vi "Array Sizer.vi"(1 "Angular Accelerations":T1 {"Angular \nAccelerations" step=5.0}, 2 "Points out":cluster{"x":dbl, "y":dbl, "th":dbl}[](array[cluster])) -> (0 "output cluster":T1)   [LabVIEW 2019]
panel:
  # "TURN Acceleration"
  # "1"
  # "1"
  # "2"
  # "2"
  # "3"
  # "3"
  # "4"
  # "4"
  # "5"
  # "5"
  # "6"
  # "6"
  # "7"
  # "7"
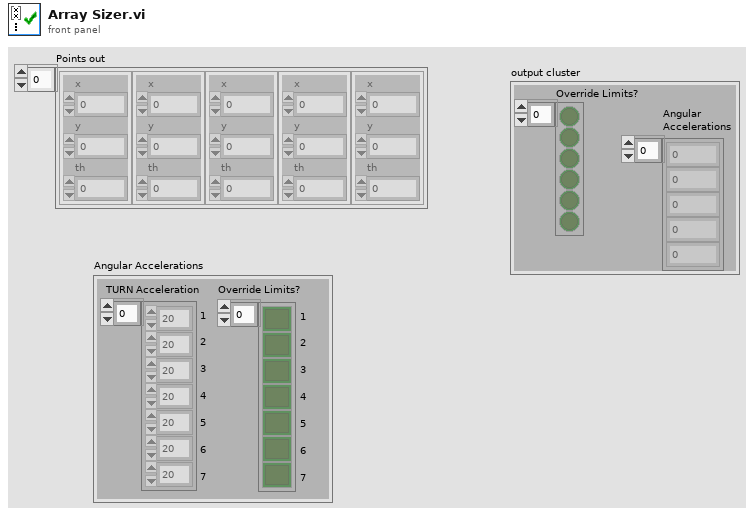
[diagram p1: front panel]
types:
  T1 = cluster{"Angular \nAccelerations":dbl[], "Override Limits?":bool[]}
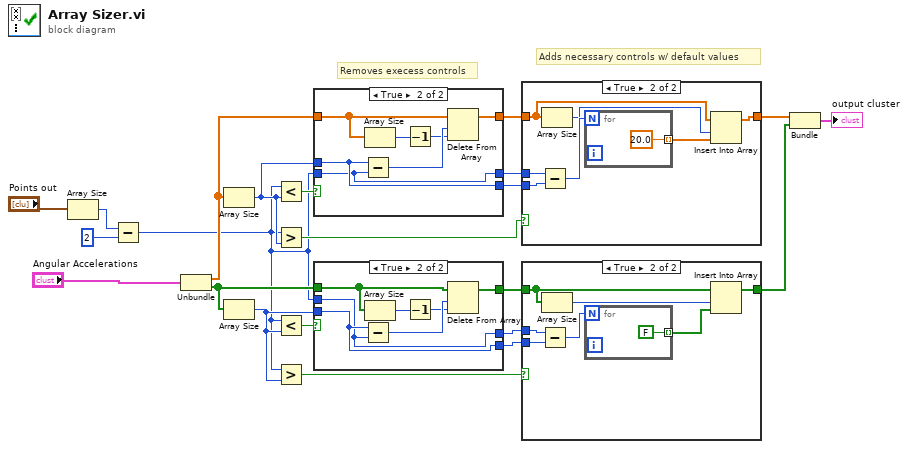
[diagram p0: block diagram]
diagram:
  # "Adds necessary controls w/ default values"
  # "Removes execess controls"
  n1 = Array Size(array="Points out") -> (size(s)=w4:i32)
  n2 = Subtract(x=w4, y=2) -> (x-y=w2:i32)
  n3 = Unbundle("Angular Accelerations") -> ("Angular \nAccelerations"=w18:dbl[], "Override Limits?"=w11:bool[])
  n4 = Array Size(array=w18) -> (size(s)=w17:i32)
  n5 = Array Size(array=w11) -> (size(s)=w10:i32)
  n6 = Less?(x=w2, y=w17) -> (x < y?=w21:bool)
  n7 = Greater?(x=w2, y=w17) -> (0:w20:bool)
  n8 = Less?(x=w2, y=w10) -> (x < y?=w5:bool)
  n9 = Greater?(x=w2, y=w10) -> (0:w6:bool)
  n10 = case shown="True" w21 {
    tunnel: [w25 w26] -> w19
    tunnel: w18 -> [w25 w29]
    tunnel: w2 -> [w24 w31]
    tunnel: w17 -> [w23 w32]
    tunnel: [w24 w31] -> w16
    tunnel: [w23 w32] -> w15
    frame False {
    }
    frame True {
      n11 = Subtract(x=w32, y=w31) -> (x-y=w30:i32)
      n12 = Array Size(array=w29) -> (size(s)=w28:i32)
      n13 = Decrement(x=w28) -> (x-1=w27:i32)
      n14 = Delete From Array(array=w29, length=w30, index=w27) -> (array with subset deleted=w26:dbl[])  [unwired: 1 out]
    }
  }
  n15 = case shown="True" w5 {
    tunnel: [w35 w36] -> w12
    tunnel: w11 -> [w35 w39]
    tunnel: w2 -> [w34 w41]
    tunnel: w10 -> [w33 w42]
    tunnel: [w34 w41] -> w13
    tunnel: [w33 w42] -> w14
    frame False {
    }
    frame True {
      n16 = Subtract(x=w42, y=w41) -> (x-y=w40:i32)
      n17 = Array Size(array=w39) -> (size(s)=w38:i32)
      n18 = Decrement(x=w38) -> (x-1=w37:i32)
      n19 = Delete From Array(array=w39, length=w40, index=w37) -> (array with subset deleted=w36:bool[])  [unwired: 1 out]
    }
  }
  n20 = case shown="True" w20 {
    tunnel: [w43 w47] -> w9
    tunnel: w19 -> [w43 w46]
    tunnel: w16 -> [_ w50]
    tunnel: w15 -> [_ w49]
    frame False {
    }
    frame True {
      n21 = Subtract(x=w50, y=w49) -> (x-y=w48:i32)
      n22 = Array Size(array=w46) -> (size(s)=w45:i32)
      n23 = for {
        N: w48 -> [_]
        tunnel: [20.0] -> w44 mode=indexing
      }
      n24 = Insert Into Array(array=w46, index=w45, new element=w44) -> (w47:dbl[])
    }
  }
  n25 = case shown="True" w6 {
    tunnel: [w52 w56] -> w8
    tunnel: w12 -> [w52 w55]
    tunnel: w13 -> [_ w59]
    tunnel: w14 -> [_ w58]
    frame False {
    }
    frame True {
      n26 = Subtract(x=w59, y=w58) -> (x-y=w57:i32)
      n27 = Array Size(array=w55) -> (size(s)=w54:i32)
      n28 = for {
        N: w57 -> [_]
        tunnel: [FALSE] -> w53 mode=indexing
      }
      n29 = Insert Into Array(array=w55, index=w54, new element=w53) -> (w56:bool[])
    }
  }
  n30 = Bundle("Angular \nAccelerations"=w9, "Override Limits?"=w8) -> (→"output cluster":T1)  [unwired: 1 in]
